vi "Sort_Channel_Map.vi"(1 "Channels map":T1[](array[typedef])) -> (0 "Sorted Channels map":T1[](array[typedef]))   [LabVIEW 2021]
uses:
  Channel_Cluster.ctl
  776d60be-e6e8-4e5a-9e51-e66961cd1bf5.vi
  <vilib>/Comparison/Less/Less Functor/Less Functor.lvclass
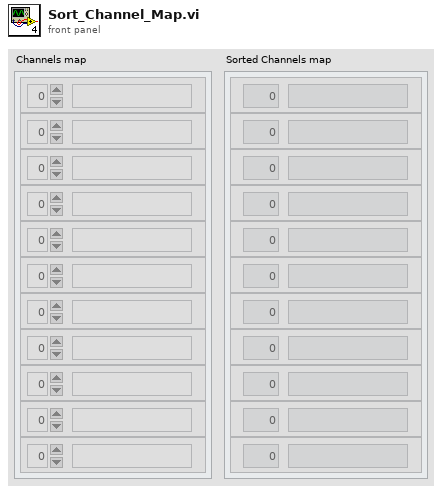
[diagram p1: front panel]
types:
  T1 = typedef "Channel_Cluster.ctl" = cluster{"Channel name":string, "Channel":u8}
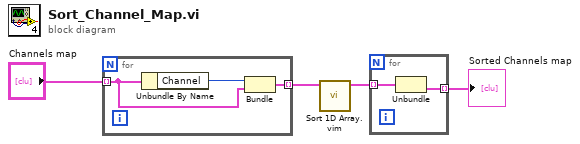
[diagram p0: block diagram]
diagram:
  n1 = for {
    tunnel: "Channels map" -> [w6] mode=indexing
    tunnel: [w5] -> w3 mode=indexing
    n2 = Unbundle By Name(w6) -> ("Channel"=w7:u8)
    n3 = Bundle("Channel"=w7, "Channel Cluster"=w6) -> (w5:cluster{"Channel":u8, "Channel Cluster":T1})  [unwired: 1 in]
  }
  n4 = call "Sort 1D Array.vim"("unsorted array"=w3) -> ("sorted array"=w2:cluster{"Channel":u8, "Channel Cluster":T1}[])  [unwired: 10 in]
  n5 = for {
    tunnel: w2 -> [w9] mode=indexing
    tunnel: [w8] -> w1 mode=indexing
    n6 = Unbundle(w9) -> ("Channel Cluster"=w8:T1)  [unwired: 1 out]
  }
  "Sorted Channels map" <- w1
